vi "ShooterStateMachine.vi"(0 "Shoot Button":bool, 1 "FeederSpeedDemand":dbl, 2 "ShooterSpeedDemand":dbl, 5 "ShooterSpeedThreshold":dbl, 7 "Rev Button":bool, 9 "Target Shooter Speed":dbl, 11 "BeltSpeedDemand":dbl, 12 "State":i32) -> (4 "ShooterSpeed":dbl, 6 "FeederSpeed":dbl, 8 "BeltSpeed":dbl, 15 "NextState":i32)   [LabVIEW 2020]
uses:
  AuxGlobals.vi
  <vilib>/Utility/semaphor.llb/Obtain Semaphore Reference.vi
  <vilib>/Rock Robotics/WPI/ThirdParty/JAS_Junk/TrajLib/Timer_Reset.vi
  <vilib>/Rock Robotics/WPI/ThirdParty/JAS_Junk/TrajLib/Trajectory_Library.lvlib
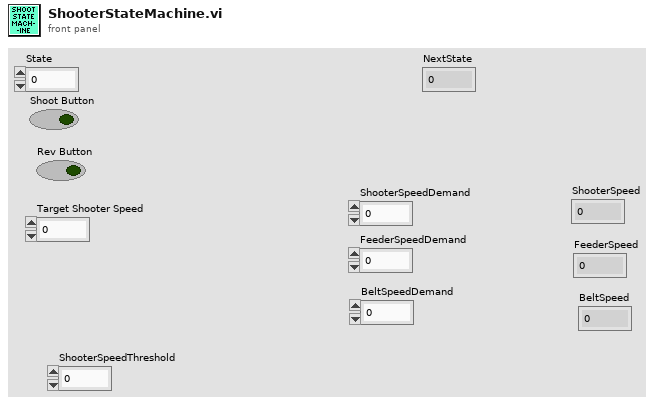
[diagram p1: front panel]
types:
  T1 = typedef "Trajectory_Library.lvlib/TIMER.ctl" = cluster{"StartTime":dbl, "Accumulated TIme":dbl, "Running":bool, "semaphore":T2}
  T2 = typedef "Semaphore RefNum" = refnum<k1>
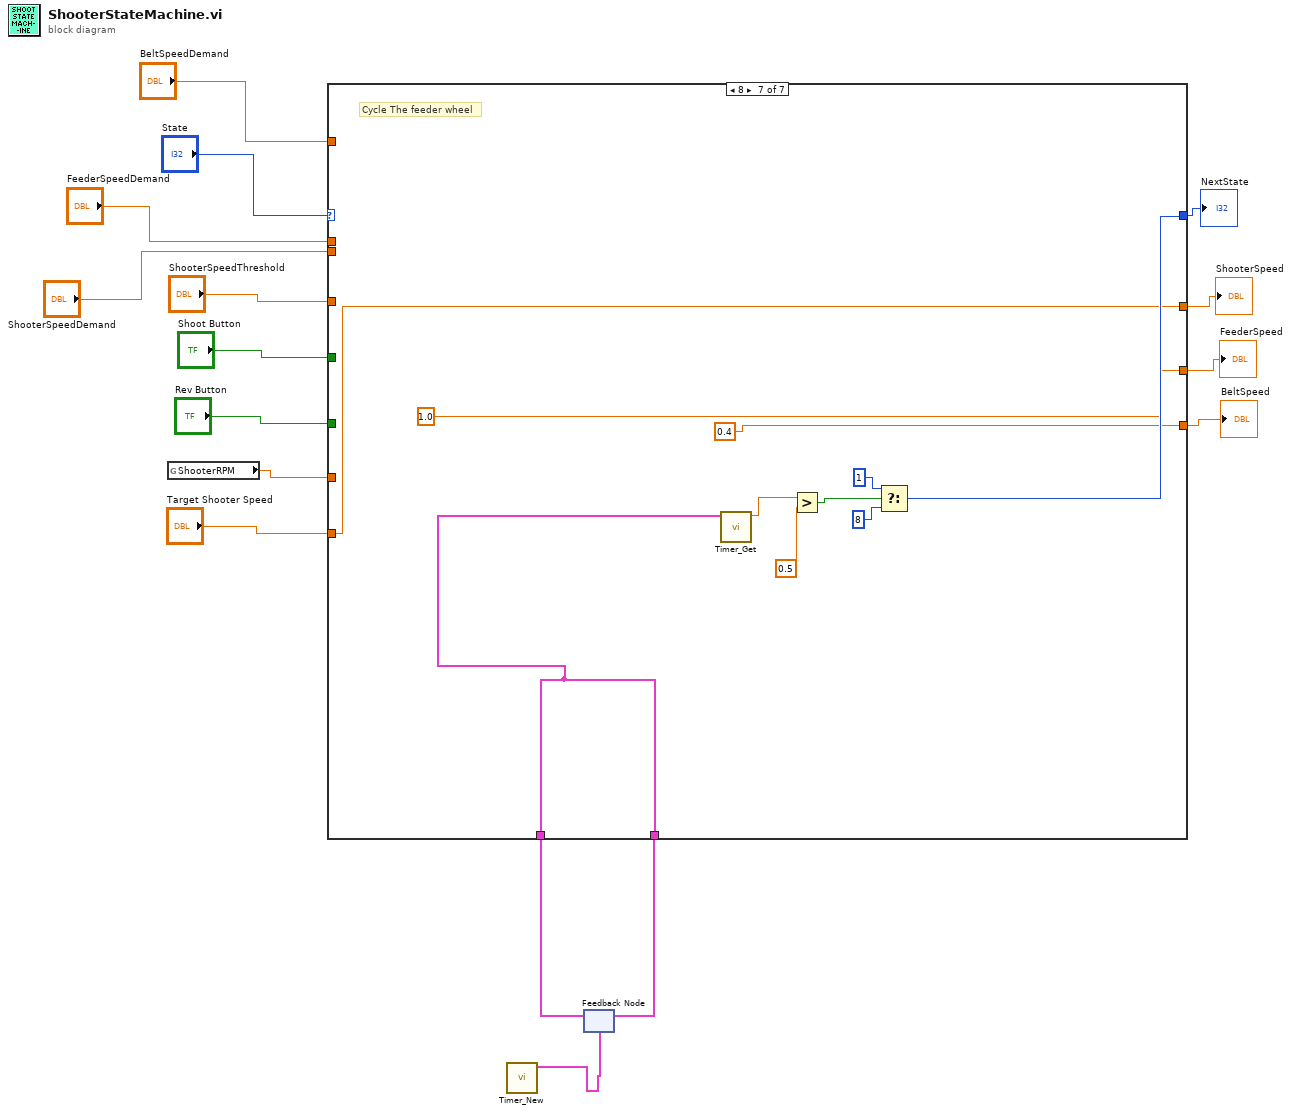
[diagram p0: block diagram]
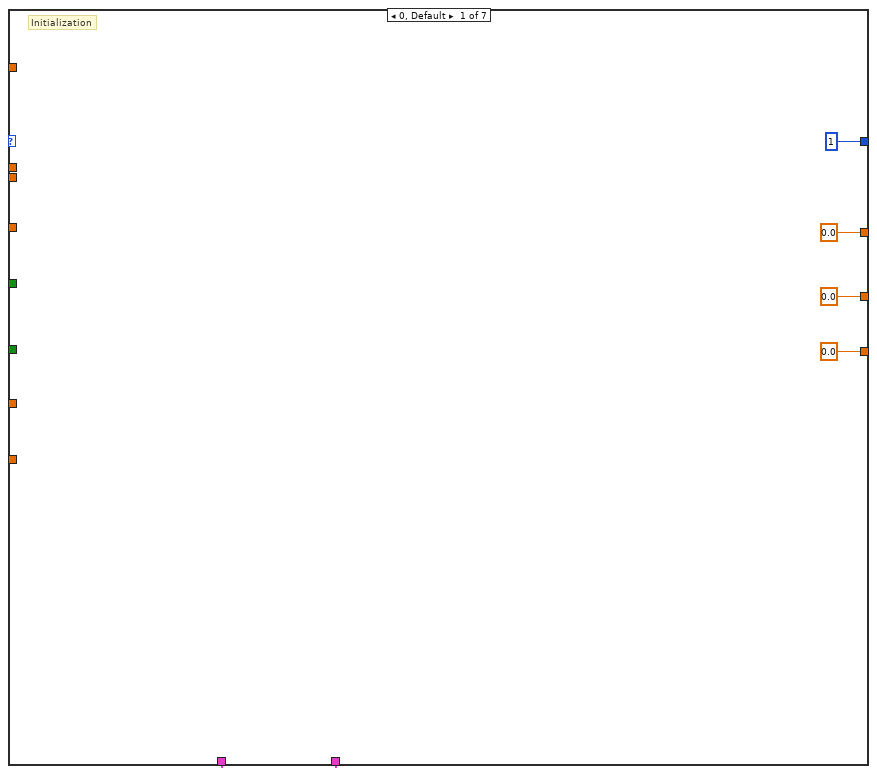
[diagram p2: hidden frame]
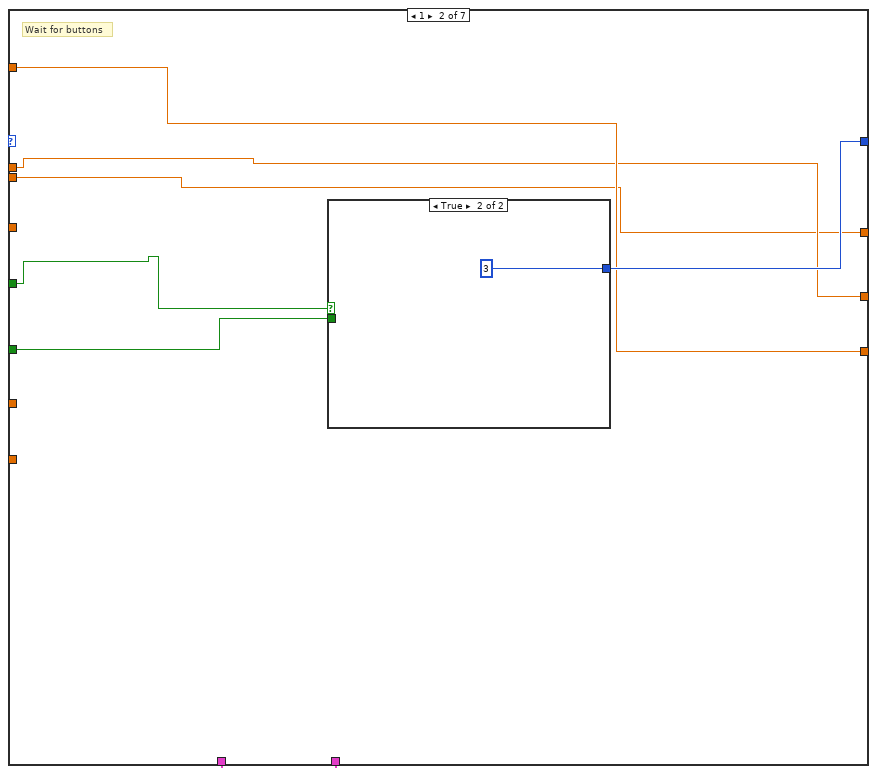
[diagram p3: hidden frame]
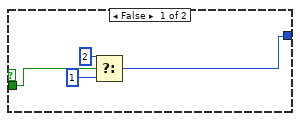
[diagram p4: hidden frame]
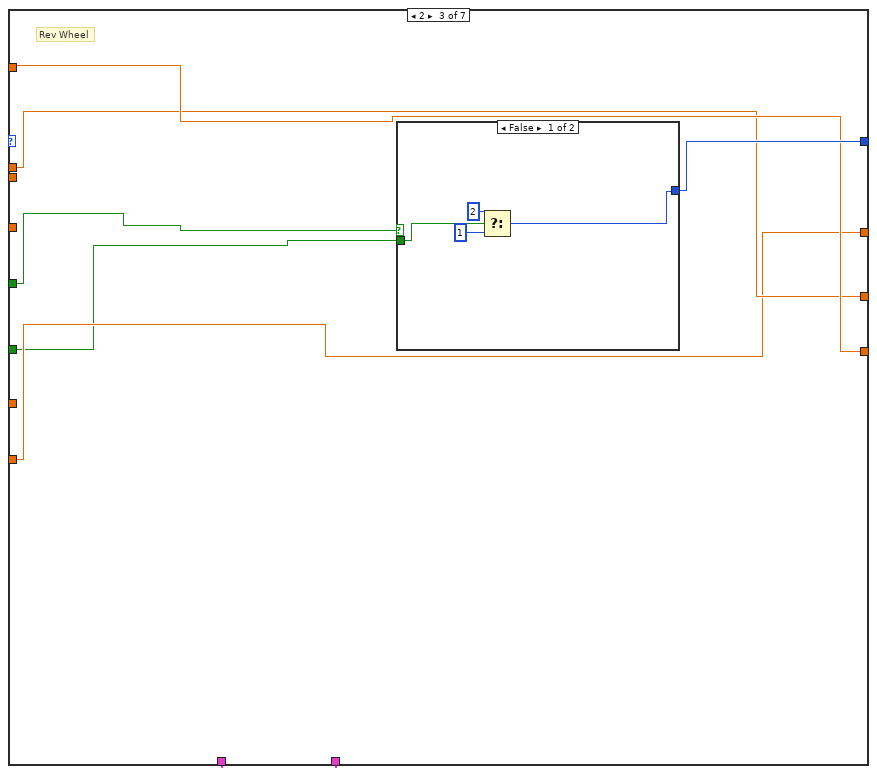
[diagram p5: hidden frame]
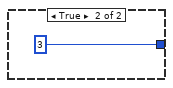
[diagram p6: hidden frame]
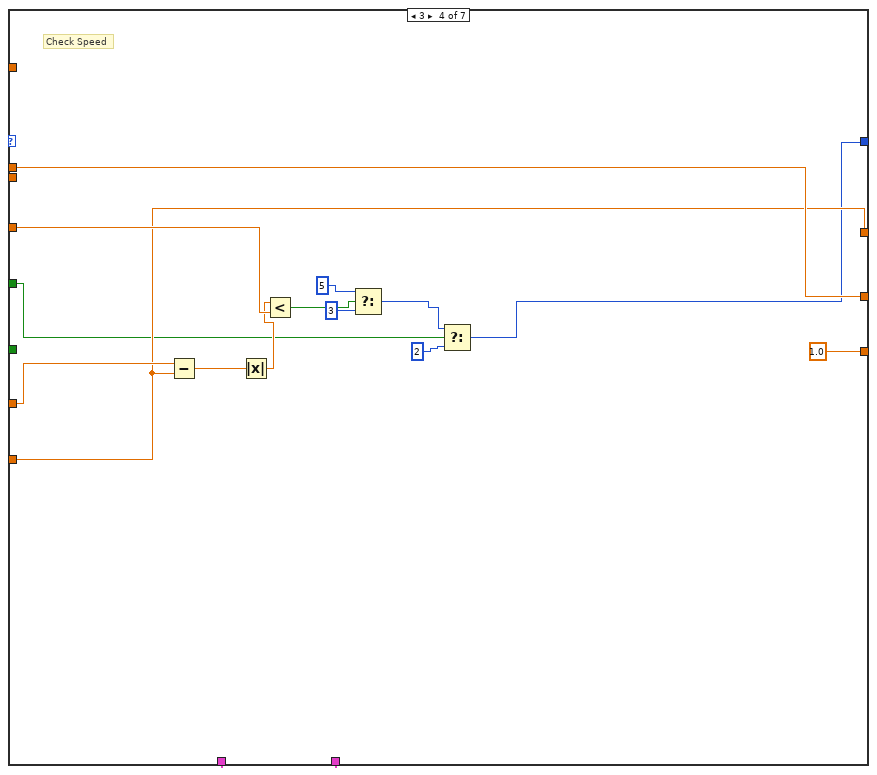
[diagram p7: hidden frame]
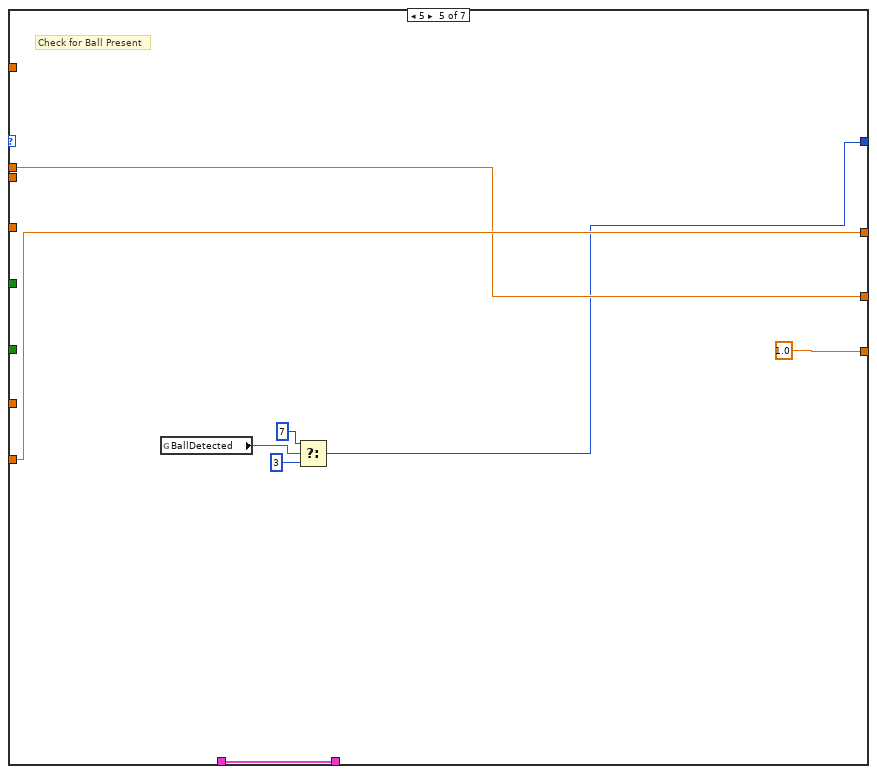
[diagram p8: hidden frame]
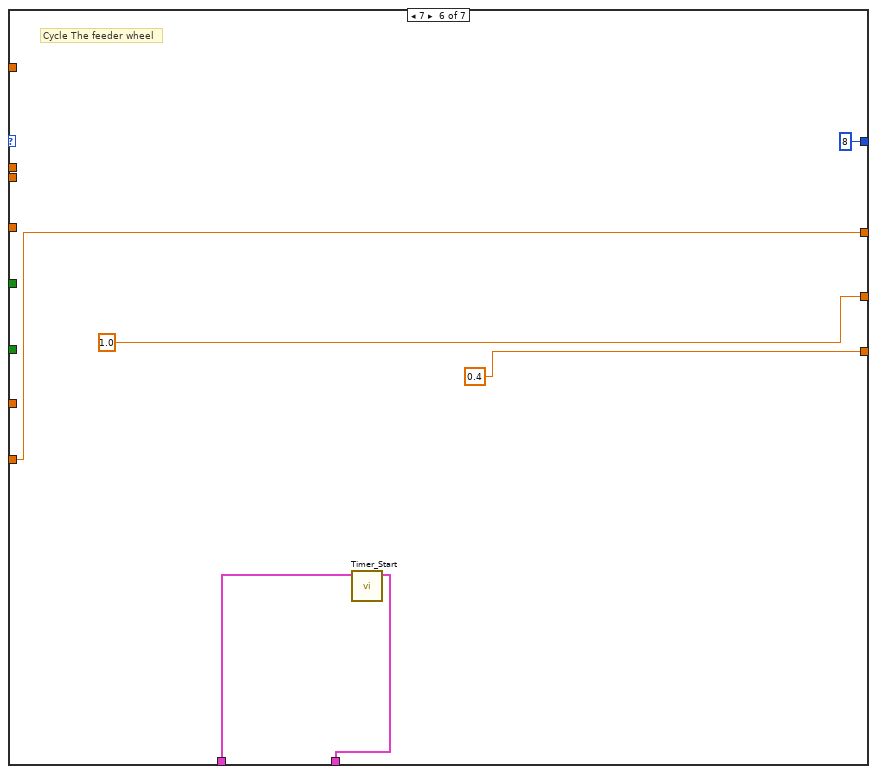
[diagram p9: hidden frame]
diagram:
  n1 = global read "AuxGlobals.vi" "ShooterRPM"() -> (w12:dbl)
  n2 = call <vilib>:"Timer_New.vi"() -> ("TIMER"=w1:T1)  [unwired: 11 in]
  n3 = feedback #1(w1) -> (w2:T1)
  n4 = case shown="8" "State" {
    tunnel: [1 w28 w40 w47 w66 8 ("f") w82] -> w15
    tunnel: "Rev Button" -> [_ w23 w35 _ _ _ _]
    tunnel: "Shoot Button" -> [_ w22 w34 w46 _ _ _]
    tunnel: w12 -> [_ _ _ w60 _ _ _]
    tunnel: "Target Shooter Speed" -> [_ _ w37 w53 w68 w73 w78]
    tunnel: "ShooterSpeedThreshold" -> [_ _ _ w57 _ _ _]
    tunnel: "BeltSpeedDemand" -> [_ w27 w39 _ _ _ _]
    tunnel: "FeederSpeedDemand" -> [_ w26 w38 w54 w67 _ _]
    tunnel: "ShooterSpeedDemand" -> [_ w25 _ _ _ _ _]
    tunnel: [0.0 ("BeltSpeedDemand") w27 w39 1.0 ("BeltSpeedDemand") 1.0 ("BeltSpeedDemand") 0.4 ("BeltSpeedDemand") 0.4 ("BeltSpeedDemand")] -> w6
    tunnel: [0.0 ("FeederSpeedDemand") w26 w38 w54 w67 1.0 ("FeederSpeedDemand") 1.0 ("FeederSpeedDemand")] -> w5
    tunnel: [0.0 ("ShooterSpeedDemand") w25 w37 w53 w68 w73 w78] -> w4
    tunnel: [w17 w24 w36 w52 w61 w70 w76] -> w3
    tunnel: w2 -> [w17 w24 w36 w52 w61 w71 w76]
    frame 0, Default {
      # "Initialization"
    }
    frame 1 {
      # "Wait for buttons"
      n5 = case shown="True" w22 {
        tunnel: [w29 3] -> w28
        tunnel: w23 -> [w32 _]
        frame False {
          n6 = Select(t=2, s=w32, f=1) -> (s? t:f=w29:i32)
        }
        frame True {
        }
      }
    }
    frame 2 {
      # "Rev Wheel"
      n7 = case shown="False" w34 {
        tunnel: [w41 3] -> w40
        tunnel: w35 -> [w44 _]
        frame False {
          n8 = Select(t=2, s=w44, f=1) -> (s? t:f=w41:i32)
        }
        frame True {
        }
      }
    }
    frame 3 {
      # "Check Speed"
      n9 = Subtract(x=w60, y=w53) -> (x-y=w59:dbl)
      n10 = Absolute Value(x=w59) -> (abs(x)=w56:dbl)
      n11 = Less?(x=w56, y=w57) -> (x < y?=w58:bool)
      n12 = Select(t=5, s=w58, f=3) -> (s? t:f=w48:i32)
      n13 = Select(t=w48, s=w46, f=2) -> (s? t:f=w47:i32)
    }
    frame 5 {
      # "Check for Ball Present"
      n14 = global read "AuxGlobals.vi" "BallDetected"() -> (w63:bool)
      n15 = Select(t=7, s=w63, f=3) -> (s? t:f=w66:i32)
    }
    frame 7 {
      # "Cycle The feeder wheel"
      n16 = call <vilib>:"Timer_Start.vi"("in Timer"=w71) -> ("out Timer"=w70:T1)  [unwired: 10 in]
    }
    frame 8 {
      # "Cycle The feeder wheel"
      n17 = call <vilib>:"Timer_Get.vi"("TIMER"=w76) -> ("CurrentTImer"=w77:dbl)  [unwired: 10 in]
      n18 = Greater?(x=w77, y=0.5) -> (0:w81:bool)
      n19 = Select(t=1, s=w81, f=8) -> (s? t:f=w82:i32)
    }
  }
  "NextState" <- w15
  "BeltSpeed" <- w6
  "FeederSpeed" <- w5
  "ShooterSpeed" <- w4
  n20 = feedback-in #1(w3) -> ()
